vi "Invalid Response.vi"(7 "error source vi name":string, 8 "error in (no error)":errorcluster, 9 "actual response":T1, 10 "expected response":T1, 11 "Dispatcher Interface in":refnum<class "Dispatcher Interface.lvclass">) -> (0 "error out":errorcluster, 3 "Dispatcher Interface out":refnum<class "Dispatcher Interface.lvclass">)   [LabVIEW 2017, in "DSF Core.lvlib" / "Dispatcher Interface.lvclass"]
uses:
  Dispatcher Interface.lvclass
  Response.ctl
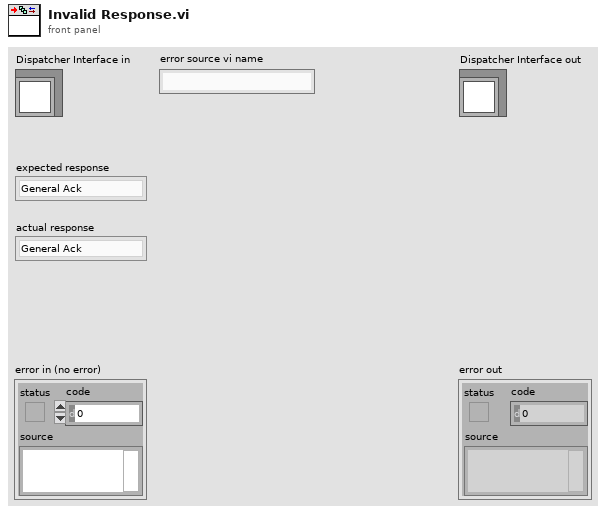
[diagram p1: front panel]
types:
  T1 = typedef "DSF Core.lvlib/Dispatcher Interface.lvclass/Response.ctl" = enum8{"General Ack", "Error", "Shutting Down"}
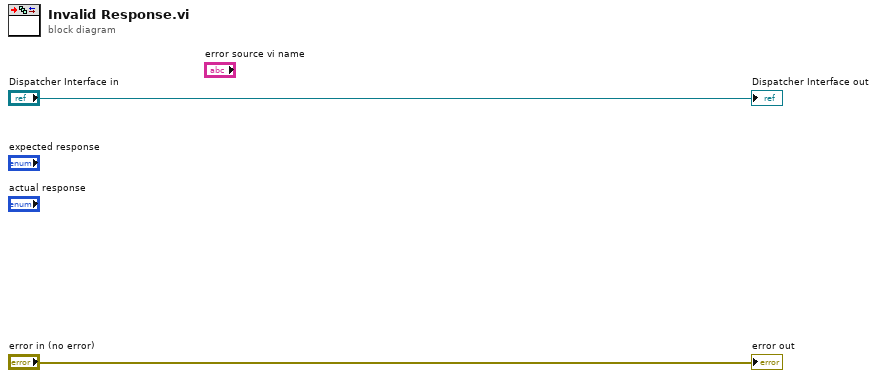
[diagram p0: block diagram]
diagram:
  "error out" <- "error in (no error)"
  "Dispatcher Interface out" <- "Dispatcher Interface in"
